vi "Build Rules.vi"() -> ()   [LabVIEW 2013]
uses:
  <vilib>/xml/Close Reference(Node).vi
  <vilib>/xml/NI_XML.lvlib
  <resource>/objmgr/DOMUserDefRef.rc
panel:
  in  "Error String":string
  in  "Save XML":bool
  in  "Generate XML":bool
  in  "Delete Rule":bool
  in  "Multicolumn Listbox":i32(listbox)
  out "Constraints.xml":string
  in  "Submit Rule":bool
  in  "stop":bool
  in  "Insert":bool
  in  "Type":enum16{"Boolean", "Numeric"}(ring)
  in  "New Rule":string
  in  "Variable":u16(ring) items=["Supply Truck On Yellow", "Evac Sign Upright", "Cargo Plane", "Tree Branch Below Wires", "All Waves On Mat", "Ambulance In Yellow", "Runway Clear", "Construction Relocation", "Base Isolation", "Code Construction", "Obstacles", "Progress", "Family", "Safety- People In Red", "Safety- People In Yellow", "Pets", "Water", "Supplies- In Red", "Supplies- In Yellow", "Safe Place", "Penalties- Outside Light Blue", "Penalties- Inside Light Blue"]
  out "Array":cluster{"Name":string, "Options":string[]}[](array[cluster])
  in  "Elements File Path":path
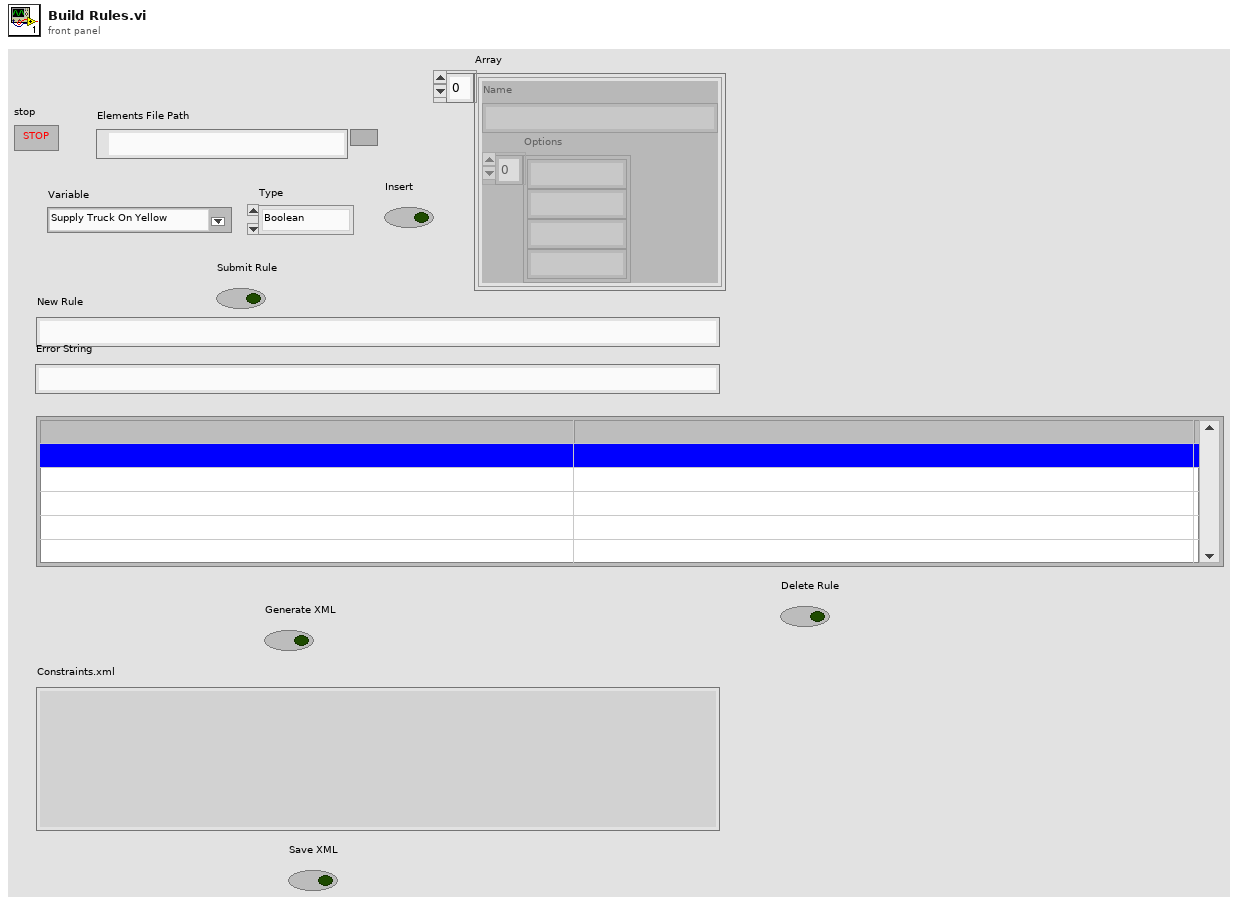
[diagram p1: front panel]
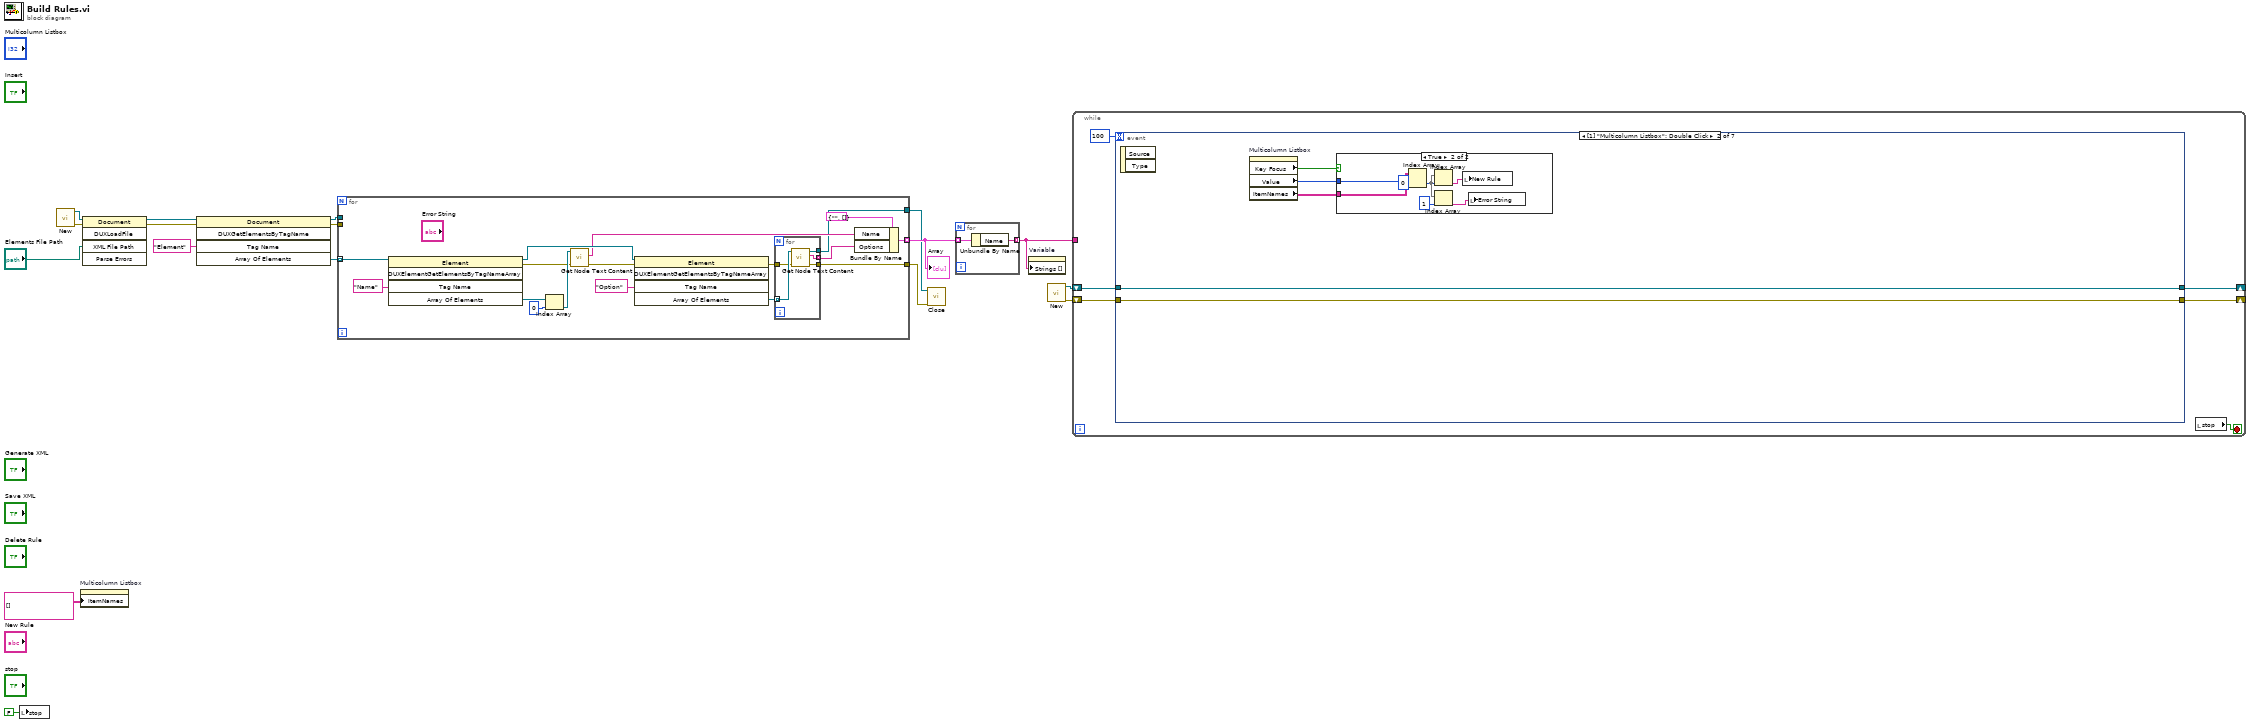
[diagram p0: block diagram]
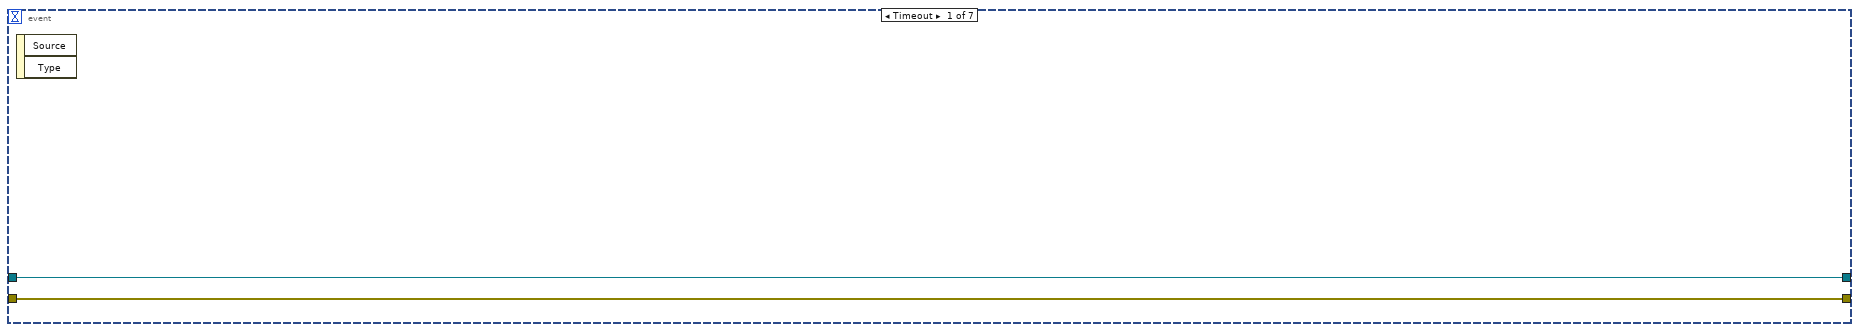
[diagram p2: hidden frame]
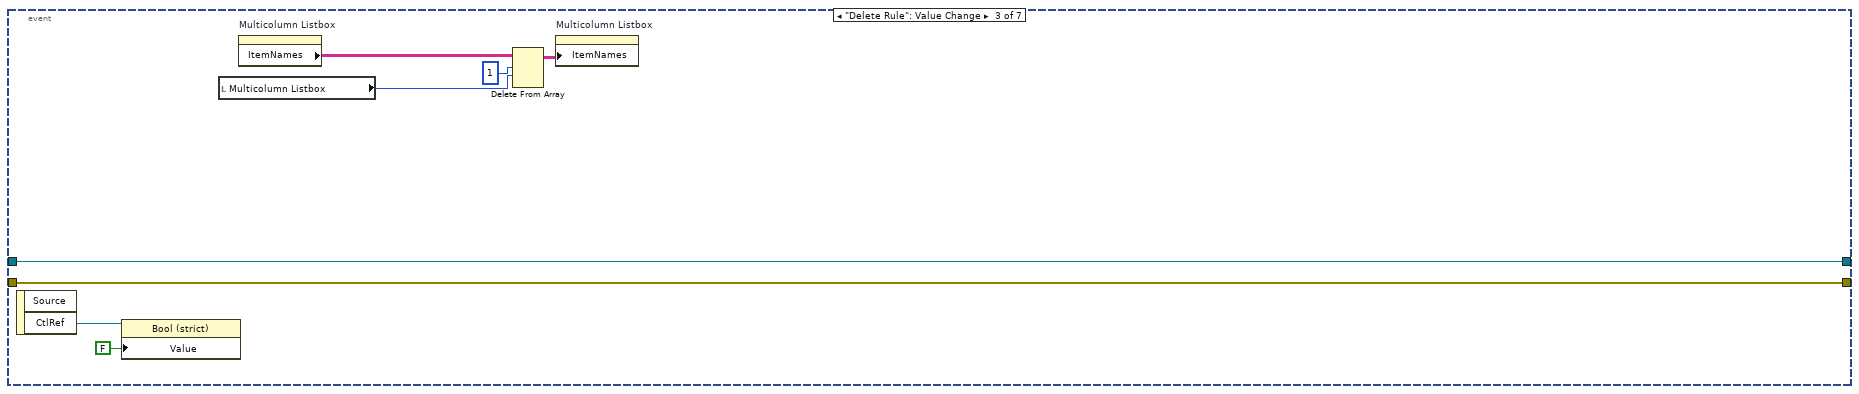
[diagram p4: hidden frame]
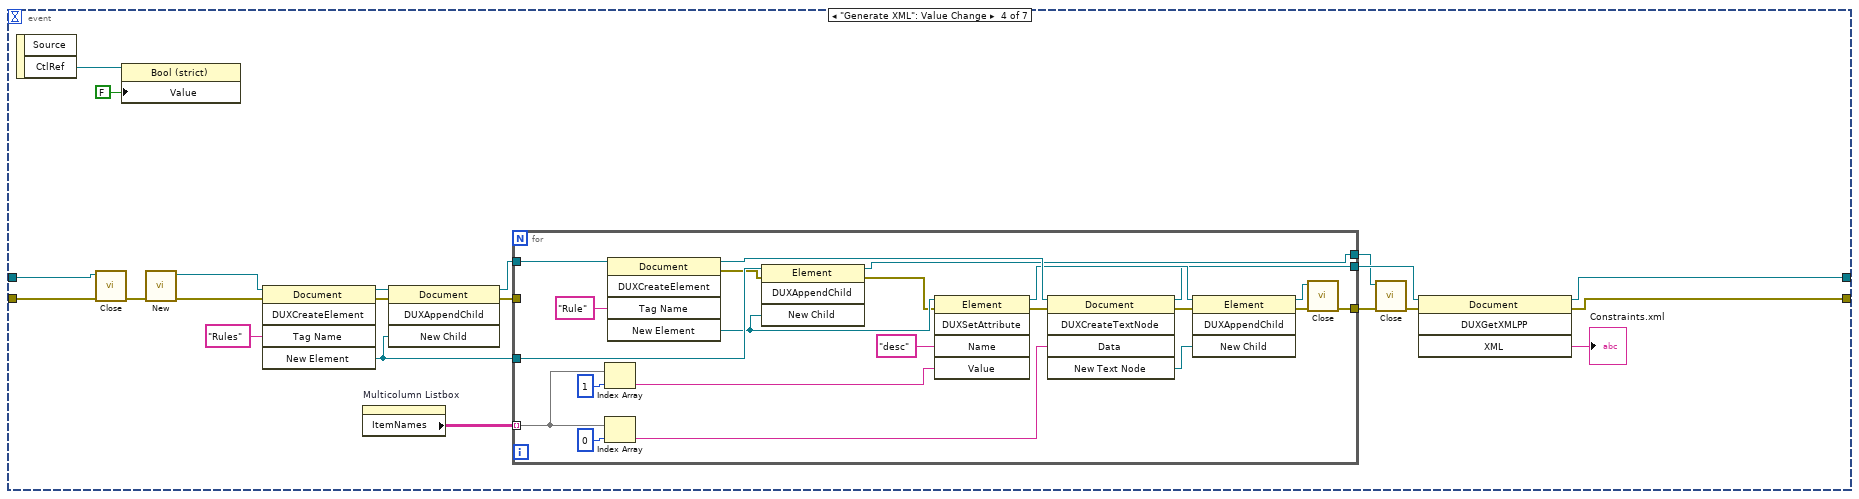
[diagram p5: hidden frame]
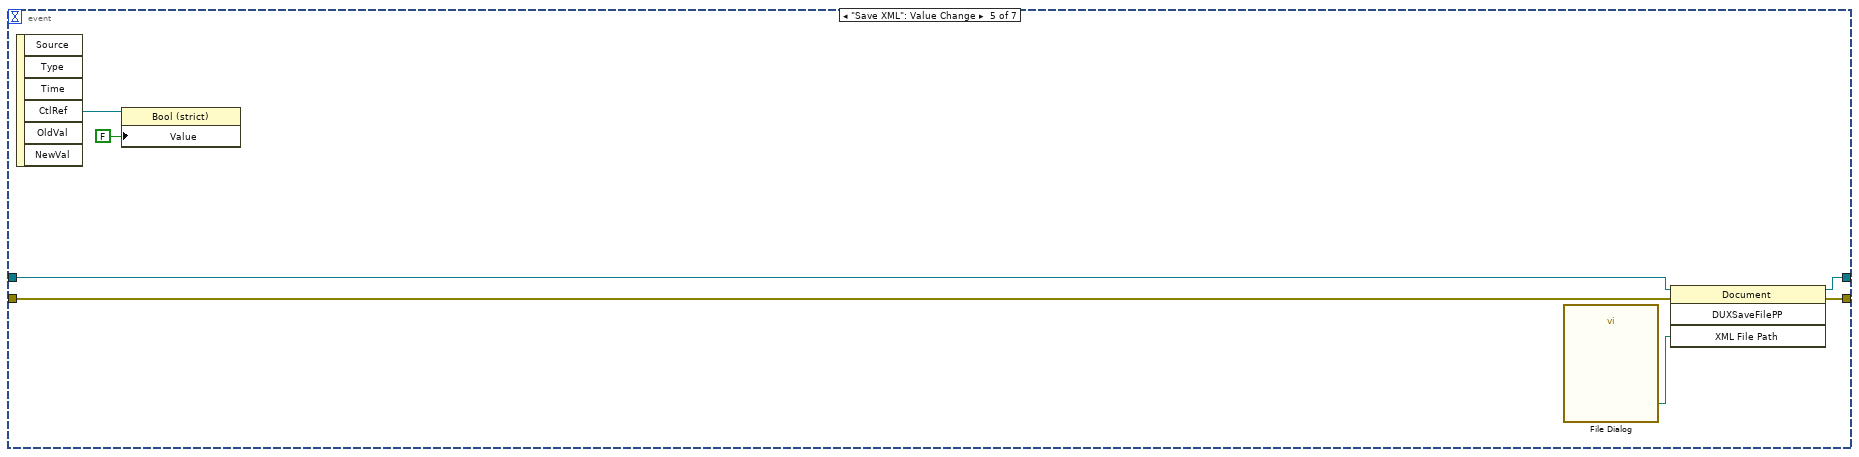
[diagram p6: hidden frame]
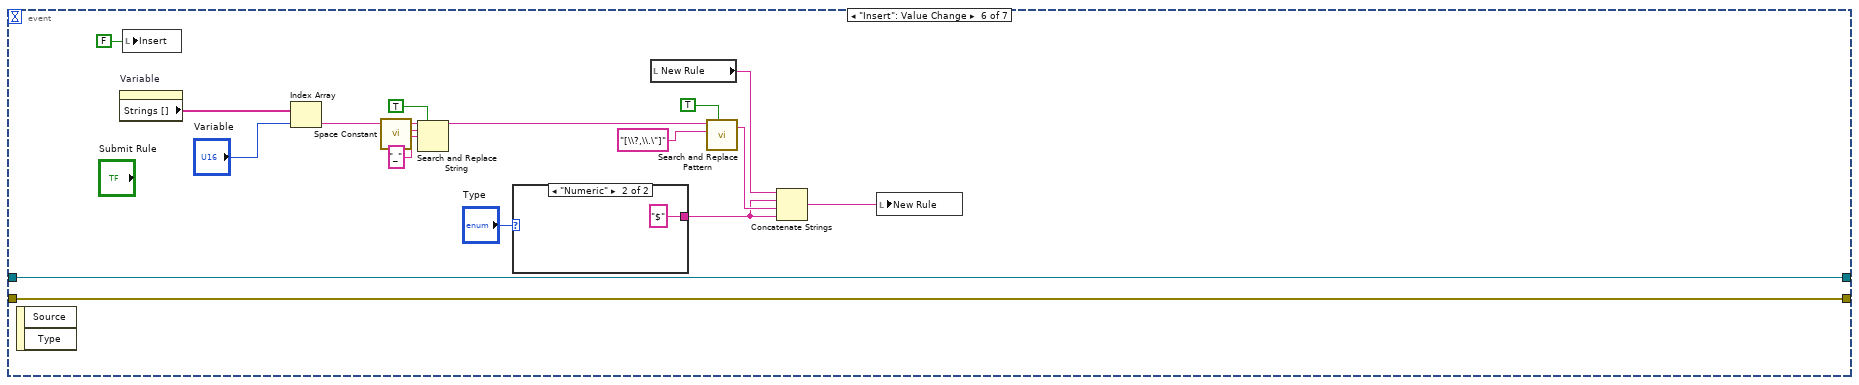
[diagram p7: hidden frame]
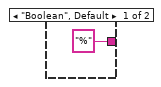
[diagram p8: hidden frame]
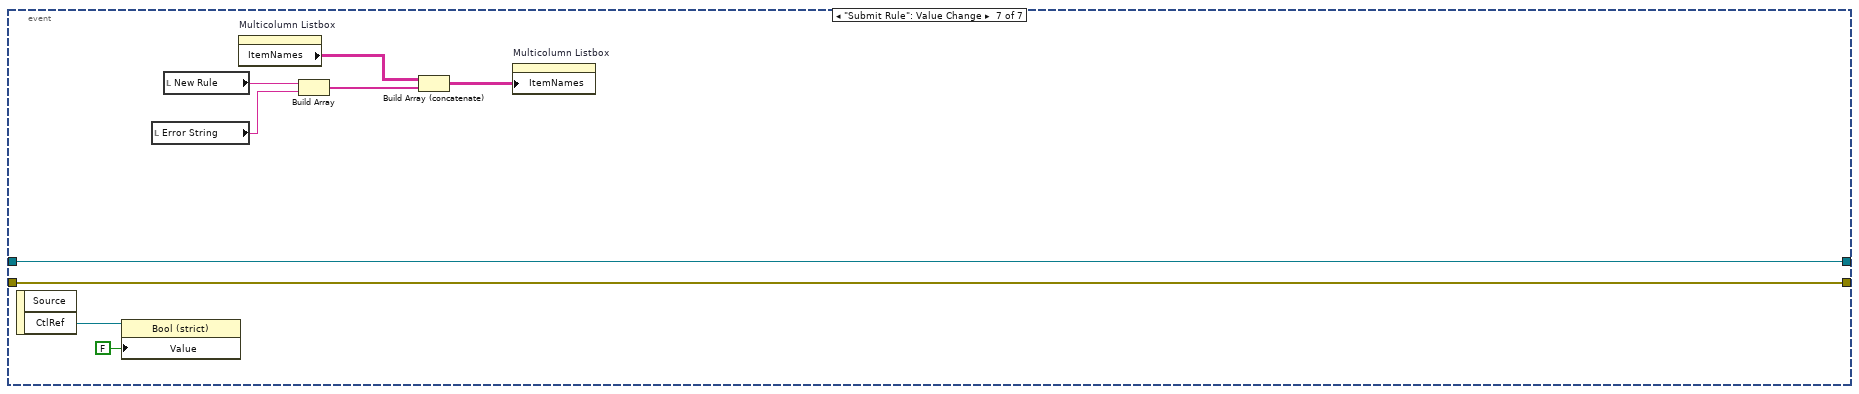
[diagram p9: hidden frame]
diagram:
  n1 = local write "stop"(FALSE ("stop")) -> ()
  n2 = call <vilib>:"New.vi"() -> ("error out"=w16:errorcluster, "DOM document out"=w17:refnum<k20>)  [unwired: 8 in]
  n3 = property on="Multicolumn Listbox" class="MCListbox (strict)"("ItemNames"=string[][] []) -> ()  [unwired: 2 in, 2 out]
  n4 = invoke class="Document" method="DUXLoadFile"(reference=w17, error in=w16, "XML File Path"="Elements File Path") -> (reference out=w14:refnum<k20>, error out=w13:errorcluster)  [unwired: 2 in, 3 out]
  n5 = invoke class="Document" method="DUXGetElementsByTagName"(reference=w14, error in=w13, "Tag Name"="Element") -> (reference out=w9:refnum<k20>, error out=w10:errorcluster, "Array Of Elements"=w11:refnum<k20>[])  [unwired: 2 in, 2 out]
  n6 = for {
    tunnel: w11 -> [w34] mode=indexing
    tunnel: w10 -> [_]
    tunnel: w9 -> [_]
    tunnel: [w20] -> w8 mode=indexing
    tunnel: [w19] -> w6
    tunnel: [w18] -> w5
    n7 = invoke class="Element" method="DUXElementGetElementsByTagNameArray"(reference=w34, "Tag Name"="Name") -> (reference out=w28:refnum<k20>, error out=w29:errorcluster, "Array Of Elements"=w32:refnum<k20>[])  [unwired: 3 in, 2 out]
    n8 = Index Array(array=w32, index=0) -> (element=w30:refnum<k20>)
    n9 = call <vilib>:"Get Node Text Content.vi"("error in (no error)"=w29, "node in"=w30) -> ("error out"=w27:errorcluster, "node text"=w21:string)  [unwired: 7 in, 1 out]
    n10 = invoke class="Element" method="DUXElementGetElementsByTagNameArray"(reference=w28, error in=w27, "Tag Name"="Option") -> (error out=w24:errorcluster, "Array Of Elements"=w25:refnum<k20>[])  [unwired: 2 in, 3 out]
    n11 = for {
      tunnel: w25 -> [w39] mode=indexing
      tunnel: w24 -> [w38]
      tunnel: [w37] -> w22 mode=indexing
      tunnel: [w36] -> w19
      tunnel: [w35] -> w18
      n12 = call <vilib>:"Get Node Text Content.vi"("error in (no error)"=w38, "node in"=w39) -> ("error out"=w35:errorcluster, "node text"=w37:string, "node out"=w36:refnum<k20>)  [unwired: 7 in]
    }
    n13 = Bundle By Name(cluster=cluster{"Name":string, "Options":string[]} {"Name"="", "Options"=[]}, "Name"=w21, "Options"=w22) -> (w20:cluster{"Name":string, "Options":string[]})
  }
  "Array" <- w8
  n14 = call-poly <vilib>:"Close.vi"("error in (no error)"=w5, "node"=w6) -> ()  [unwired: 7 in, 1 out]
  n15 = for {
    tunnel: w8 -> [w41] mode=indexing
    tunnel: [w40] -> w4 mode=indexing
    n16 = Unbundle By Name(w41) -> ("Name"=w40:string)
  }
  n17 = property on="Variable" class="Ring (strict)"("Strings []"=w4) -> ()  [unwired: 2 in, 2 out]
  n18 = call <vilib>:"New.vi"() -> ("error out"=w1:errorcluster, "DOM document out"=w2:refnum<k20>)  [unwired: 8 in]
  n19 = while {
    tunnel: w4 -> [_]
    shift-right: [w42] -> _
    shift-left: w2 -> [w45]
    shift-right: [w43] -> _
    shift-left: w1 -> [w44]
    stop <- w46 stop-if-true
    n20 = event shown="[1] \"Multicolumn Listbox\": Double Click" {
      selector: _ -> [_ _ _ _ _ _ _]
      dyn-events: _ -> [_ _ _ _ _ _ _]
      timeout: 100 -> [_ _ _ _ _ _ _]
      tunnel: w45 -> [w49 w51 w65 w90 w116 w121 w146]
      tunnel: w44 -> [w48 w50 w64 w89 w115 w120 w145]
      tunnel: [w48 w50 w64 w74 w117 w120 w145] -> w43
      tunnel: [w49 w51 w65 w75 w118 w121 w146] -> w42
      event Timeout {
        n21 = event-data() -> ()  [unwired: 1 in, 2 out]
      }
      event "Multicolumn Listbox": Double Click {
        n22 = event-data() -> ()  [unwired: 1 in, 2 out]
        n23 = property on="Multicolumn Listbox" class="MCListbox (strict)"() -> ("Key Focus"=w54:bool, "Value"=w53:i32, "ItemNames"=w52:string[][])  [unwired: 2 in, 2 out]
        n24 = case shown="True" w54 {
          tunnel: w53 -> [_ w60]
          tunnel: w52 -> [_ w61]
          frame False {
          }
          frame True {
            n25 = Index Array(array=w61, index (row)=w60) -> (element=w57:string[])  [unwired: 1 in]
            n26 = Index Array(array=w57, index=1) -> (element=w55:string)
            n27 = Index Array(array=w57, index=0) -> (element=w58:string)
            n28 = local write "New Rule"(w58) -> ()
            n29 = local write "Error String"(w55) -> ()
          }
        }
      }
      event "Delete Rule": Value Change {
        n30 = event-data() -> ("CtlRef"=w62:refnum<vi>)  [unwired: 1 in, 1 out]
        n31 = property class="Bool (strict)"(reference=w62, "Value"=FALSE) -> ()  [unwired: 1 in, 2 out]
        n32 = local read "Multicolumn Listbox"() -> (w68:i32)
        n33 = property on="Multicolumn Listbox" class="MCListbox (strict)"() -> ("ItemNames"=w67:string[][])  [unwired: 2 in, 2 out]
        n34 = Delete From Array(array=w67, length=1, index (row)=w68) -> (array with subset deleted=w66:string[][])  [unwired: 1 in, 1 out]
        n35 = property on="Multicolumn Listbox" class="MCListbox (strict)"("ItemNames"=w66) -> ()  [unwired: 2 in, 2 out]
      }
      event "Generate XML": Value Change {
        n36 = event-data() -> ("CtlRef"=w71:refnum<vi>)  [unwired: 1 in, 1 out]
        n37 = call-poly <vilib>:"Close.vi"("error in (no error)"=w89, "node"=w90) -> ("error out"=w88:errorcluster)  [unwired: 7 in]
        n38 = property class="Bool (strict)"(reference=w71, "Value"=FALSE) -> ()  [unwired: 1 in, 2 out]
        n39 = call <vilib>:"New.vi"("error in (no error)"=w88) -> ("error out"=w86:errorcluster, "DOM document out"=w87:refnum<k20>)  [unwired: 7 in]
        n40 = invoke class="Document" method="DUXCreateElement"(reference=w87, error in=w86, "Tag Name"="Rules") -> (reference out=w84:refnum<k20>, error out=w83:errorcluster, "New Element"=w79:refnum<k20>)  [unwired: 2 in, 2 out]
        n41 = property on="Multicolumn Listbox" class="MCListbox (strict)"() -> ("ItemNames"=w82:string[][])  [unwired: 2 in, 2 out]
        n42 = invoke class="Document" method="DUXAppendChild"(reference=w84, error in=w83, "New Child"=w79) -> (reference out=w81:refnum<k20>, error out=w80:errorcluster)  [unwired: 1 in, 2 out]
        n43 = for {
          tunnel: w82 -> [w102] mode=indexing
          tunnel: w81 -> [w112]
          tunnel: w80 -> [_]
          tunnel: w79 -> [w110]
          tunnel: [w94] -> w78
          tunnel: [w93] -> w77
          tunnel: [w92] -> w70
          n44 = Index Array(array=w102, index=1) -> (element=w106:string)
          n45 = Index Array(array=w102, index=0) -> (element=w100:string)
          n46 = invoke class="Document" method="DUXCreateElement"(reference=w112, "Tag Name"="Rule") -> (reference out=w103:refnum<k20>, error out=w109:errorcluster, "New Element"=w105:refnum<k20>)  [unwired: 3 in, 2 out]
          n47 = invoke class="Element" method="DUXAppendChild"(reference=w110, error in=w109, "New Child"=w105) -> (reference out=w92:refnum<k20>, error out=w104:errorcluster)  [unwired: 1 in, 2 out]
          n48 = invoke class="Element" method="DUXSetAttribute"(reference=w105, error in=w104, "Name"="desc", "Value"=w106) -> (reference out=w99:refnum<k20>, error out=w98:errorcluster)  [unwired: 1 in, 3 out]
          n49 = invoke class="Document" method="DUXCreateTextNode"(reference=w103, error in=w98, "Data"=w100) -> (reference out=w93:refnum<k20>, error out=w97:errorcluster, "New Text Node"=w91:refnum<k20>)  [unwired: 2 in, 2 out]
          n50 = invoke class="Element" method="DUXAppendChild"(reference=w99, error in=w97, "New Child"=w91) -> (reference out=w96:refnum<k20>, error out=w95:errorcluster)  [unwired: 1 in, 2 out]
          n51 = call-poly <vilib>:"Close.vi"("error in (no error)"=w95, "node"=w96) -> ("error out"=w94:errorcluster)  [unwired: 7 in]
        }
        n52 = call-poly <vilib>:"Close.vi"("error in (no error)"=w78, "node"=w70) -> ("error out"=w76:errorcluster)  [unwired: 7 in]
        n53 = invoke class="Document" method="DUXGetXMLPP"(reference=w77, error in=w76) -> (reference out=w75:refnum<k20>, error out=w74:errorcluster, "XML"=→"Constraints.xml":string)  [unwired: 2 in, 1 out]
      }
      event "Save XML": Value Change {
        n54 = event-data() -> ("CtlRef"=w114:refnum<vi>)  [unwired: 1 in, 5 out]
        n55 = property class="Bool (strict)"(reference=w114, "Value"=FALSE) -> ()  [unwired: 1 in, 2 out]
        n56 = call "File Dialog"() -> ("selected path"=w119:path)  [unwired: 12 in, 3 out]
        n57 = invoke class="Document" method="DUXSaveFilePP"(reference=w116, error in=w115, "XML File Path"=w119) -> (reference out=w118:refnum<k20>, error out=w117:errorcluster)  [unwired: 1 in, 2 out]
      }
      event "Insert": Value Change {
        n58 = event-data() -> ()  [unwired: 1 in, 2 out]
        n59 = property on="Variable" class="Ring (strict)"() -> ("Strings []"=w136:string[])  [unwired: 2 in, 2 out]
        n60 = local write "Insert"(FALSE ("Insert")) -> ()
        n61 = Index Array(array=w136, index="Variable") -> (element=w132:string)
        n62 = call <vilib>:"Space Constant.vi"() -> ("String"=w131:string)
        n63 = Search and Replace String(replace all?=TRUE ("replace all? (F)"), input string=w132, search string=w131, replace string="_" ("replace string (\"\")")) -> (result string=w128:string)  [unwired: 4 in, 3 out]
        n64 = case shown="\"Numeric\"" "Type" {
          tunnel: ["%" "$"] -> w123
          frame "Boolean", Default {
          }
          frame "Numeric" {
          }
        }
        n65 = local read "New Rule"() -> (w134:string)
        n66 = call <vilib>:"Search and Replace Pattern.vi"("string"=w128, "regular expression (\"\")"="[\\?,\\.\"]" ("regular expression (\"\")"), "replace all? (F)"=TRUE) -> ("result string"=w125:string)  [unwired: 2 in, 1 out]
        n67 = Concatenate Strings(w134, w123, w125, w123) -> (w133:string)
        n68 = local write "New Rule"(w133) -> ()
      }
      event "Submit Rule": Value Change {
        n69 = event-data() -> ("CtlRef"=w143:refnum<vi>)  [unwired: 1 in, 1 out]
        n70 = property class="Bool (strict)"(reference=w143, "Value"=FALSE) -> ()  [unwired: 1 in, 2 out]
        n71 = local read "Error String"() -> (w140:string)
        n72 = local read "New Rule"() -> (w141:string)
        n73 = property on="Multicolumn Listbox" class="MCListbox (strict)"() -> ("ItemNames"=w142:string[][])  [unwired: 2 in, 2 out]
        n74 = Build Array(w141, w140) -> (w139:string[])
        n75 = Build Array (concatenate)(w142, w139) -> (w147:string[][])
        n76 = property on="Multicolumn Listbox" class="MCListbox (strict)"("ItemNames"=w147) -> ()  [unwired: 2 in, 2 out]
      }
    }
    n77 = local read "stop"() -> (w46:bool)
  }
